vi "Blit Surface (Wrap).vi"(6 "Destination Rectangle":T1, 7 "Use Clip (F)":bool, 8 "error in":errorcluster, 9 "Source Rectangle":T1, 10 "Destination Pointer":u32, 11 "Source Pointer":u32) -> (0 "error out":errorcluster, 3 "Return":i32)   [LabVIEW 2015]
uses:
  Controls/Rectangle.ctl
  DLL/SDL2.dll
  LibSDL2.lvlib
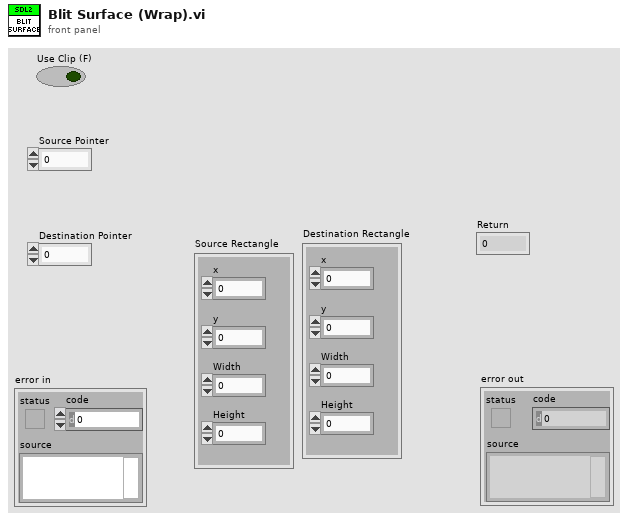
[diagram p1: front panel]
types:
  T1 = typedef "LibSDL2.lvlib/Rectangle.ctl" = cluster{"x":i32, "y":i32, "Width":i32, "Height":i32}
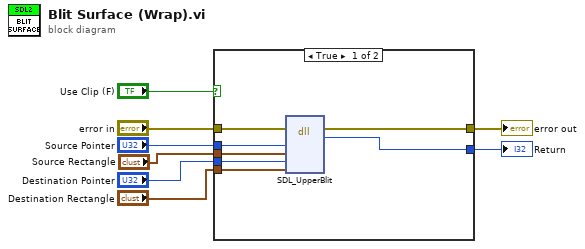
[diagram p0: block diagram]
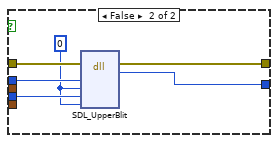
[diagram p2: hidden frame]
diagram:
  n1 = case shown="True" "Use Clip (F)" {
    tunnel: "error in" -> [w15 w21]
    tunnel: [w14 w20] -> w7
    tunnel: "Source Pointer" -> [w13 w19]
    tunnel: "Destination Pointer" -> [w12 w18]
    tunnel: [w11 w17] -> w4
    tunnel: "Destination Rectangle" -> [w10 _]
    tunnel: "Source Rectangle" -> [w9 _]
    frame True {
      n2 = dll-call lib="C:/dev/PGS/LabSDL2/Source/Libraries/LibSDL2 Wrapper/DLL/SDL2.dll" fn="SDL_UpperBlit"(error in=w15, "src"=w13, "srcrect"=w9, "dst"=w12, "dstrect"=w10) -> (error out=w14:errorcluster, "return type"=w11:i32)  [unwired: 6 in, 1 out]
    }
    frame False {
      w16 = u32 0
      n3 = dll-call lib="C:/dev/PGS/LabSDL2/Source/Libraries/LibSDL2 Wrapper/DLL/SDL2.dll" fn="SDL_UpperBlit"(error in=w21, "src"=w19, "srcrect"=w16, "dst"=w18, "dstrect"=w16) -> (error out=w20:errorcluster, "return type"=w17:i32)  [unwired: 6 in, 1 out]
    }
  }
  "error out" <- w7
  "Return" <- w4
